vi "RunWireCalibration.vi"() -> ()   [LabVIEW 2016]
uses:
  Controls/0_XYZstage/BOOL_Moving.ctl
  <vilib>/userdefined/High Color/IMAQdx.ctl
  <vilib>/Utility/miscctls.llb/LVRowAndColumnUnsignedTypeDef.ctl
  Controls/All_Enums/Enum_TypeDef_ImageSharpnessAnalysisMethod.ctl
  <vilib>/Analysis/6fits.llb/Curve Fitting Criteria.ctl
  <extravilib>/ChannelInstances/High Speed Stream-c(i32,str,c(dbl,dbl),t'IMAQ Image.ctl',t'IMAQdx.ctl')/_Read For Replicate.vi
  Miscellaneous/PixelToMicron.vi
  <extravilib>/ChannelInstances/High Speed Stream-c(i32,str,c(dbl,dbl),t'IMAQ Image.ctl',t'IMAQdx.ctl')/Instantiate.vi
  <extravilib>/ChannelInstances/High Speed Stream-c(i32,str,c(dbl,dbl),t'IMAQ Image.ctl',t'IMAQdx.ctl')/)Channel.vi
  <extravilib>/ChannelInstances/High Speed Stream-c(i32,str,c(dbl,dbl),t'IMAQ Image.ctl',t'IMAQdx.ctl')/Abort Signal/Init Signal.vi
  <vilib>/gmath/statdist.llb/st_Percentiles (scalar).vi
  <vilib>/vision/driver/NI_Vision_Acquisition_Software.lvlib
  <vilib>/Analysis/NI_AALPro.lvlib
  <vilib>/Analysis/NI_AALBase.lvlib
  <vilib>/gmath/NI_Gmath.lvlib
  <vilib>/LabVIEW Interface for Arduino/LabVIEW Interface for Arduino.lvlib
  <extravilib>/ChannelInstances/High Speed Stream-c(i32,str,c(dbl,dbl),t'IMAQ Image.ctl',t'IMAQdx.ctl').lvlib
panel:
  out "completed":bool
  out "Loops":i32
  out "Image Data":T1(array[cluster])
  in  "Mode":enum16{"Run Calibration", "View Results"}(ring)
  out "Finished":bool
  in  "Tab Control":T2(tab)
  in  "error tab":bool
  in  "cam session":T3="cam1" caption="Select Camera"
  in  "Short-distance\naxis speed":T4={"vX [mm/s]"=5.0, "vY [mm/s]"=5.0, "vZ [mm/s]"=5.0}
  in  "Long-distance\naxis speed":T4={"vX [mm/s]"=25.0, "vY [mm/s]"=12.5, "vZ [mm/s]"=5.0}
  in  "wait time":u32=2000 caption="wait (ms)"
  in  "Y position":dbl format="%#_13g"
  in  "Z position":dbl format="%#_13g"
  in  "percentile":dbl=95.0 caption="tolerance percentile" format="%#_13g"
  in  "Python":path=path "python"
  in  "Wire Diameter":dbl=90.0 caption="Wire Diameter (microns)"
  in  "Wire Height (mm)":dbl=2.5 format="%#_13g"
  in  "Image Info Results Read":path caption="Image Info Path"
  in  "Image File Results Read":bool=TRUE caption="View Images from Saved Location?"
  in  "Im. Source":T5(radio)
  out "Image Source Tab":T5(tab) caption="Warning: if you don't save the images, a new set of images must be captured to run the calibration again. Saving images allows the user to run the calibration on the same image set multiple times."
  in  "Disable auto-focus":bool caption="(only use if the camera was not adjusted since the most recent run of this VI)"
  in  "Home":bool=TRUE caption="Home first?"
  in  "Save Images":bool=TRUE caption="Save Images to File?"
  in  "Image Calibration Write":path=path "C:/Users/Aerotech/Desktop/Joel Images 8_7" caption="Image Path"
  in  "Image Overwrite":bool=TRUE caption="Overwrite existing files?"
  in  "Image Info Calibration Read":path caption="Image Info Path"
  in  "View Results":bool
  in  "Data File Read":path caption="Data File Path"
  in  "Run Calibration":bool
  in  "File Name":string="data_file.csv"
  in  "Data File Overwrite":bool caption="Overwrite existing files?"
  in  "Data File Write":path=path "C:/Users/Aerotech/Desktop" caption="Data File Path"
  in  "List of All Fits":i32(listbox)
  out "Progress":dbl(slide) caption="Progress: complete" scale=0.0..100.0
  out "Moving":T6
  in  "abort":bool
  in  "pause":bool
  out "Graph of Fit":cluster{dbl[], dbl[]}[](graph) caption="Graph of Fit for Image #79"
  in  "List of Failed Fits":i32(listbox)
  out "Image":T7(plugin-control) caption="Image #79"
  out "Fit Info":T8={"Initial Guess"={"Center (pixels)"=-1.0, "Reflectivity"=0.0}, "Params Vector"=[], "Errors"=[], "Iterations"=0, "Success"=FALSE} {"Errors" format="%#_2g"; "Params Vector" format="%#_10f"; "Initial Guess"."Center (pixels)" format="%#_16g"}
  in  "Quit":bool
  out "Re-do Necessary?":bool
  out "fails":i32 caption="Number of Failed Fits:"
  out "Tolerance":dbl=4.0 caption="95% Tolerance (microns):" format="%_2g"
  out "Confidence":dbl caption="95% Confidence Interval (microns):" format="%.5g"
  out "std. dev.":dbl caption="Standard Deviation (microns):" format="%.5g"
  out "outside tolerance":bool caption="Within Tolerance?"
  out "Histogram of Final Fit Residuals":T9(graph) caption="XY Graph"
  out "Adjusted Graph of Final Fit":cluster{dbl[], dbl[]}(graph) caption="XY Graph"
  out "queue error":errorcluster
  out "image file error":errorcluster
  out "info file error":errorcluster
  out "Image Display Error":errorcluster
  out "data file write error":errorcluster
  out "Capture Error":errorcluster caption="stage/camera error"
  # "NOTE: Click \"RUN\" to run the VI BEFORE entering the set-up parameters!!!"
  # "For runnung a new calibration"
  # "For viewing a previously run calibration"
  # "Image Files"
  # "Settings"
  # "Image Files"
  # "Data File"
  # "Data File"
  # "Center (px)"
  # "Reflectivity (ul)"
  # "Amplitude (px val^2)"
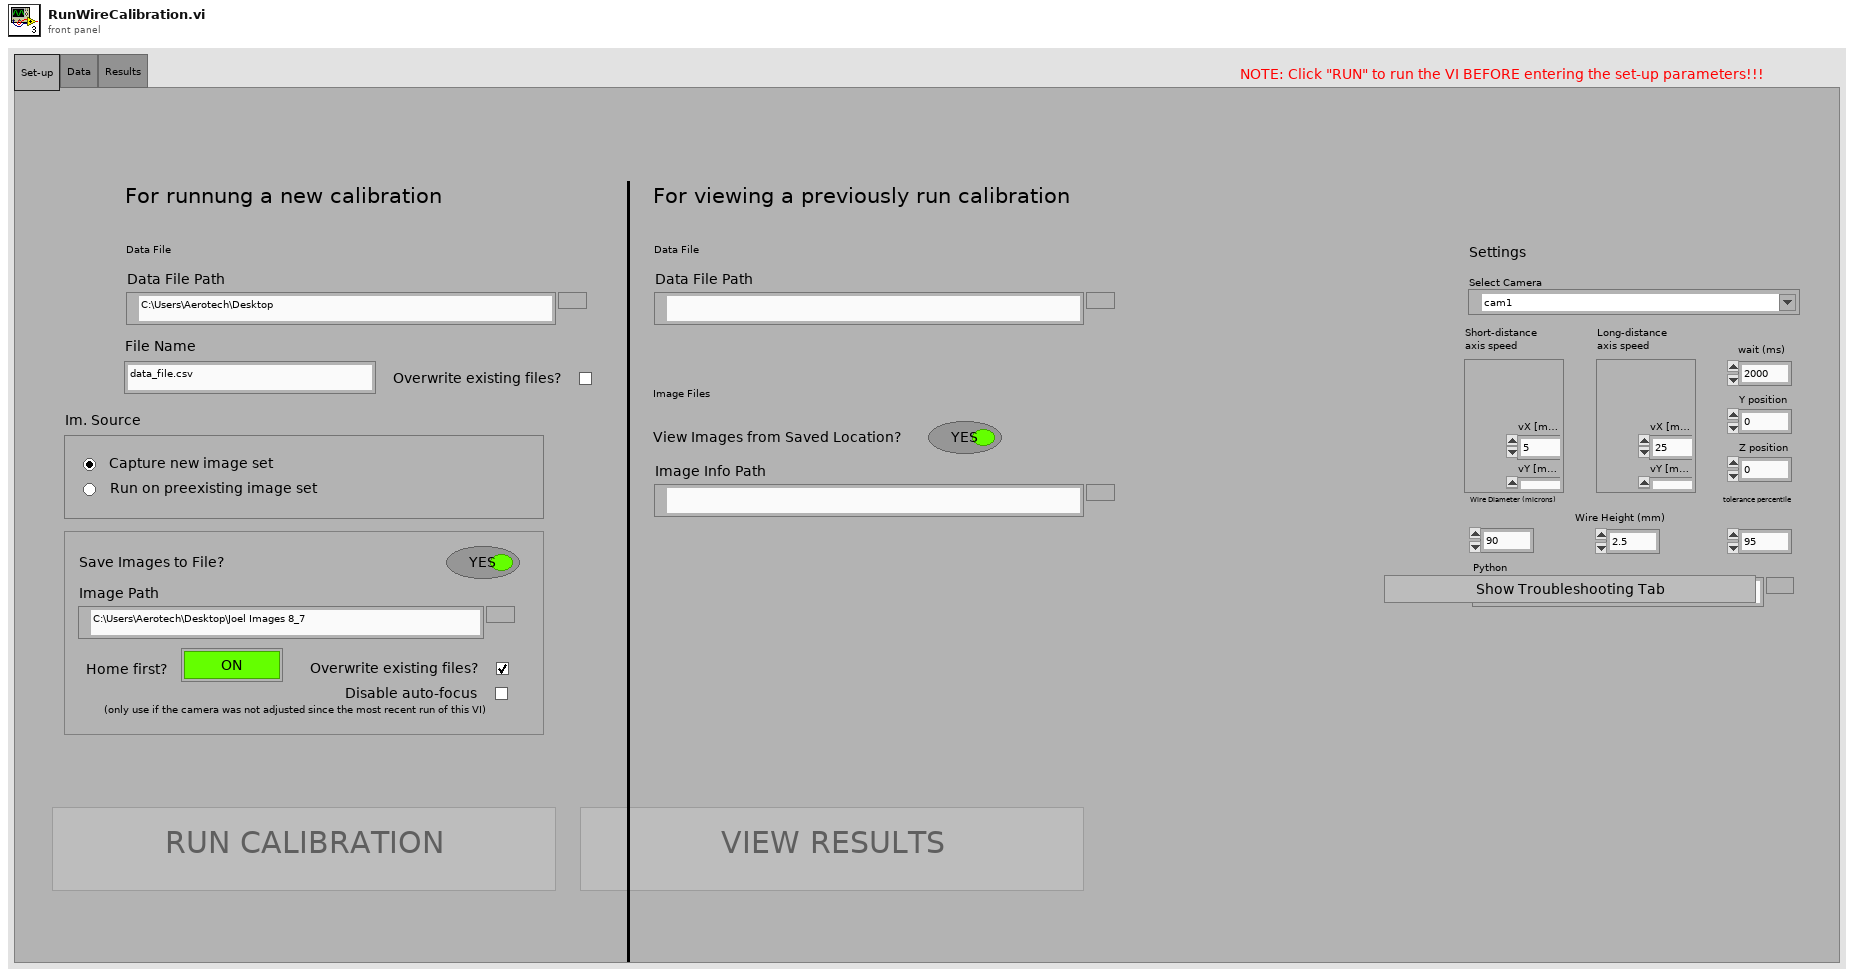
[diagram p1: front panel]
types:
  T1 = cluster{"success?":bool, "image number":i32, "camera position":cluster{"X":dbl, "Y":dbl}, "parameters":cluster{"amplitude":dbl, "center":dbl, "reflectivity":dbl}, "errors":cluster{"amplitude":dbl, "center":dbl, "reflectivity":dbl}, "Initial Guess":cluster{"center":dbl, "reflectivity":dbl}, "iterations":i32, "image path":path}[]
  T2 = enum32{"Set-up", "Data", "Results", "Troubleshooting"}
  T3 = typedef "IMAQdx.ctl" = refnum<k21>
  T4 = cluster{"vX [mm/s]":dbl, "vY [mm/s]":dbl, "vZ [mm/s]":dbl}
  T5 = enum32{"Capture new image set", "Run on preexisting image set"}
  T6 = typedef "BOOL_Moving.ctl" = bool
  T7 = typedef "IMAQ Image.ctl" = refnum<image>
  T8 = cluster{"Initial Guess":cluster{"Center (pixels)":dbl, "Reflectivity":dbl}, "Params Vector":dbl[], "Errors":dbl[], "Iterations":i32, "Success":bool}
  T9 = cluster{"X Values":dbl[], "Histogram: h(x)":i32[]}
  T10 = enum8{"Enabled", "Disabled", "Disabled and Grayed Out"}
  T11 = cluster{"Params Vector[1]":dbl, "Params Vector[2]":dbl}
  T12 = enum16{"open", "replace", "create", "open or create", "replace or create", "replace or create with confirmation"}
  T13 = cluster{"image number":i32, "image path":path, "position":cluster{dbl, dbl}}
  T14 = typedef "Enum_TypeDef_ImageSharpnessAnalysisMethod.ctl" = enum16{"sigma( Intensity )", "Mean( Laplacian Convolution )"}
  T15 = typedef "LVRowAndColumnUnsignedTypeDef.ctl" = cluster{"Row":u32, "Column":u32}
  T16 = cluster{"Data File Write":path, "File Name":string, "Data File Overwrite":bool}
  T17 = typedef "LabVIEW Interface for Arduino.lvlib/Arduino Resource.ctl" = cluster{"VISA resource":refnum<visa-resource-name>, "Board Type":T18, "Connection Type":enum8{"USB / Serial"}, "Bytes Per Packet (15)":u8}
  T18 = typedef "LabVIEW Interface for Arduino.lvlib/Board Type.ctl" = enum16{"Uno", "Dimuelanove w/Atmega 328", "Mega 2560"}
  T19 = typedef "ArduinoLT-ConfigurationControl.ctl" = cluster{"Lights: Digital I/O Pins":cluster{"Coaxial":u8, "Spotlights":u8}, "Thermistor Settings":cluster{"Analogue Readout Pin":u8, "Vcc Reference Pin":u8, "Paired Resistance (10K Ohms)":dbl, "Units (C)":enum16{"Celsius", "Fahrenheit", "Kelvin"}}}
  T20 = cluster{"Arduino Configuration OUT":T19, "Arduino Resource OUT":T17, "error out":errorcluster}
  T21 = typedef "Image Type" = u32
  T22 = cluster{"Final X":dbl, "Final Y":dbl, "Final Z":dbl}
  T23 = cluster{i32, string, cluster{"Final X":dbl, "Final Y":dbl}, "Image Out":T7, "Session Out":T3}
  T24 = typedef "High Speed Stream-c(i32,str,c(dbl,dbl),t'IMAQ Image.ctl',t'IMAQdx.ctl').lvlib/)Channel.ctl" = refnum<queue>
  T25 = cluster{"Image Calibration Write":path, "Image Overwrite":bool}
  T26 = cluster{i32, "Smart Path":path, cluster{"Final X":dbl, "Final Y":dbl}}
  T27 = cluster{i32, "appended path":path, cluster{dbl, dbl}}
  T28 = cluster{"Params Vector[0]":dbl, "Params Vector[1]":dbl, "Params Vector[2]":dbl}
  T29 = cluster{"Errors[0]":dbl, "Errors[1]":dbl, "Errors[2]":dbl}
  T30 = cluster{"Success":bool, "image number":i32, "position":cluster{dbl, dbl}, "Params Vector":cluster{"Params Vector[0]":dbl, "Params Vector[1]":dbl, "Params Vector[2]":dbl}, "Errors":cluster{"Errors[0]":dbl, "Errors[1]":dbl, "Errors[2]":dbl}, cluster{"Params Vector[1]":dbl, "Params Vector[2]":dbl}, "Iterations":i32, "image path":path}
  T31 = cluster{"Success":bool, "image number":i32, "position":cluster{"X":dbl, "Y":dbl}, "Params Vector":cluster{"Params Vector[0]":dbl, "Params Vector[1]":dbl, "Params Vector[2]":dbl}, "Errors":cluster{"Errors[0]":dbl, "Errors[1]":dbl, "Errors[2]":dbl}, "Initial Guess":cluster{"Params Vector[1]":dbl, "Params Vector[2]":dbl}, "Iterations":i32, "image path":path}[]
  T32 = cluster{bool, i32, cluster{dbl, dbl}, cluster{dbl, dbl, dbl}, cluster{dbl, dbl, dbl}, cluster{dbl, dbl}, i32, "appended path":path}
  T33 = typedef "NI_AALPro.lvlib/Curve Fitting Criteria.ctl" = u16
  T34 = cluster{"success?":bool, "image number":i32, "camera position":cluster{"X":dbl, "Y":dbl}, "parameters":cluster{"amplitude":dbl, "center":dbl, "reflectivity":dbl}, "errors":cluster{"amplitude":dbl, "center":dbl, "reflectivity":dbl}, "Initial Guess":cluster{"center":dbl, "reflectivity":dbl}, "iterations":i32, "image path":path}
  T35 = cluster{"amplitude":dbl, "center":dbl, "reflectivity":dbl}
  T36 = cluster{"Initial Guess":cluster{"center":dbl, "reflectivity":dbl}, "parameters":dbl[], "errors":dbl[], "iterations":i32, "success?":bool}
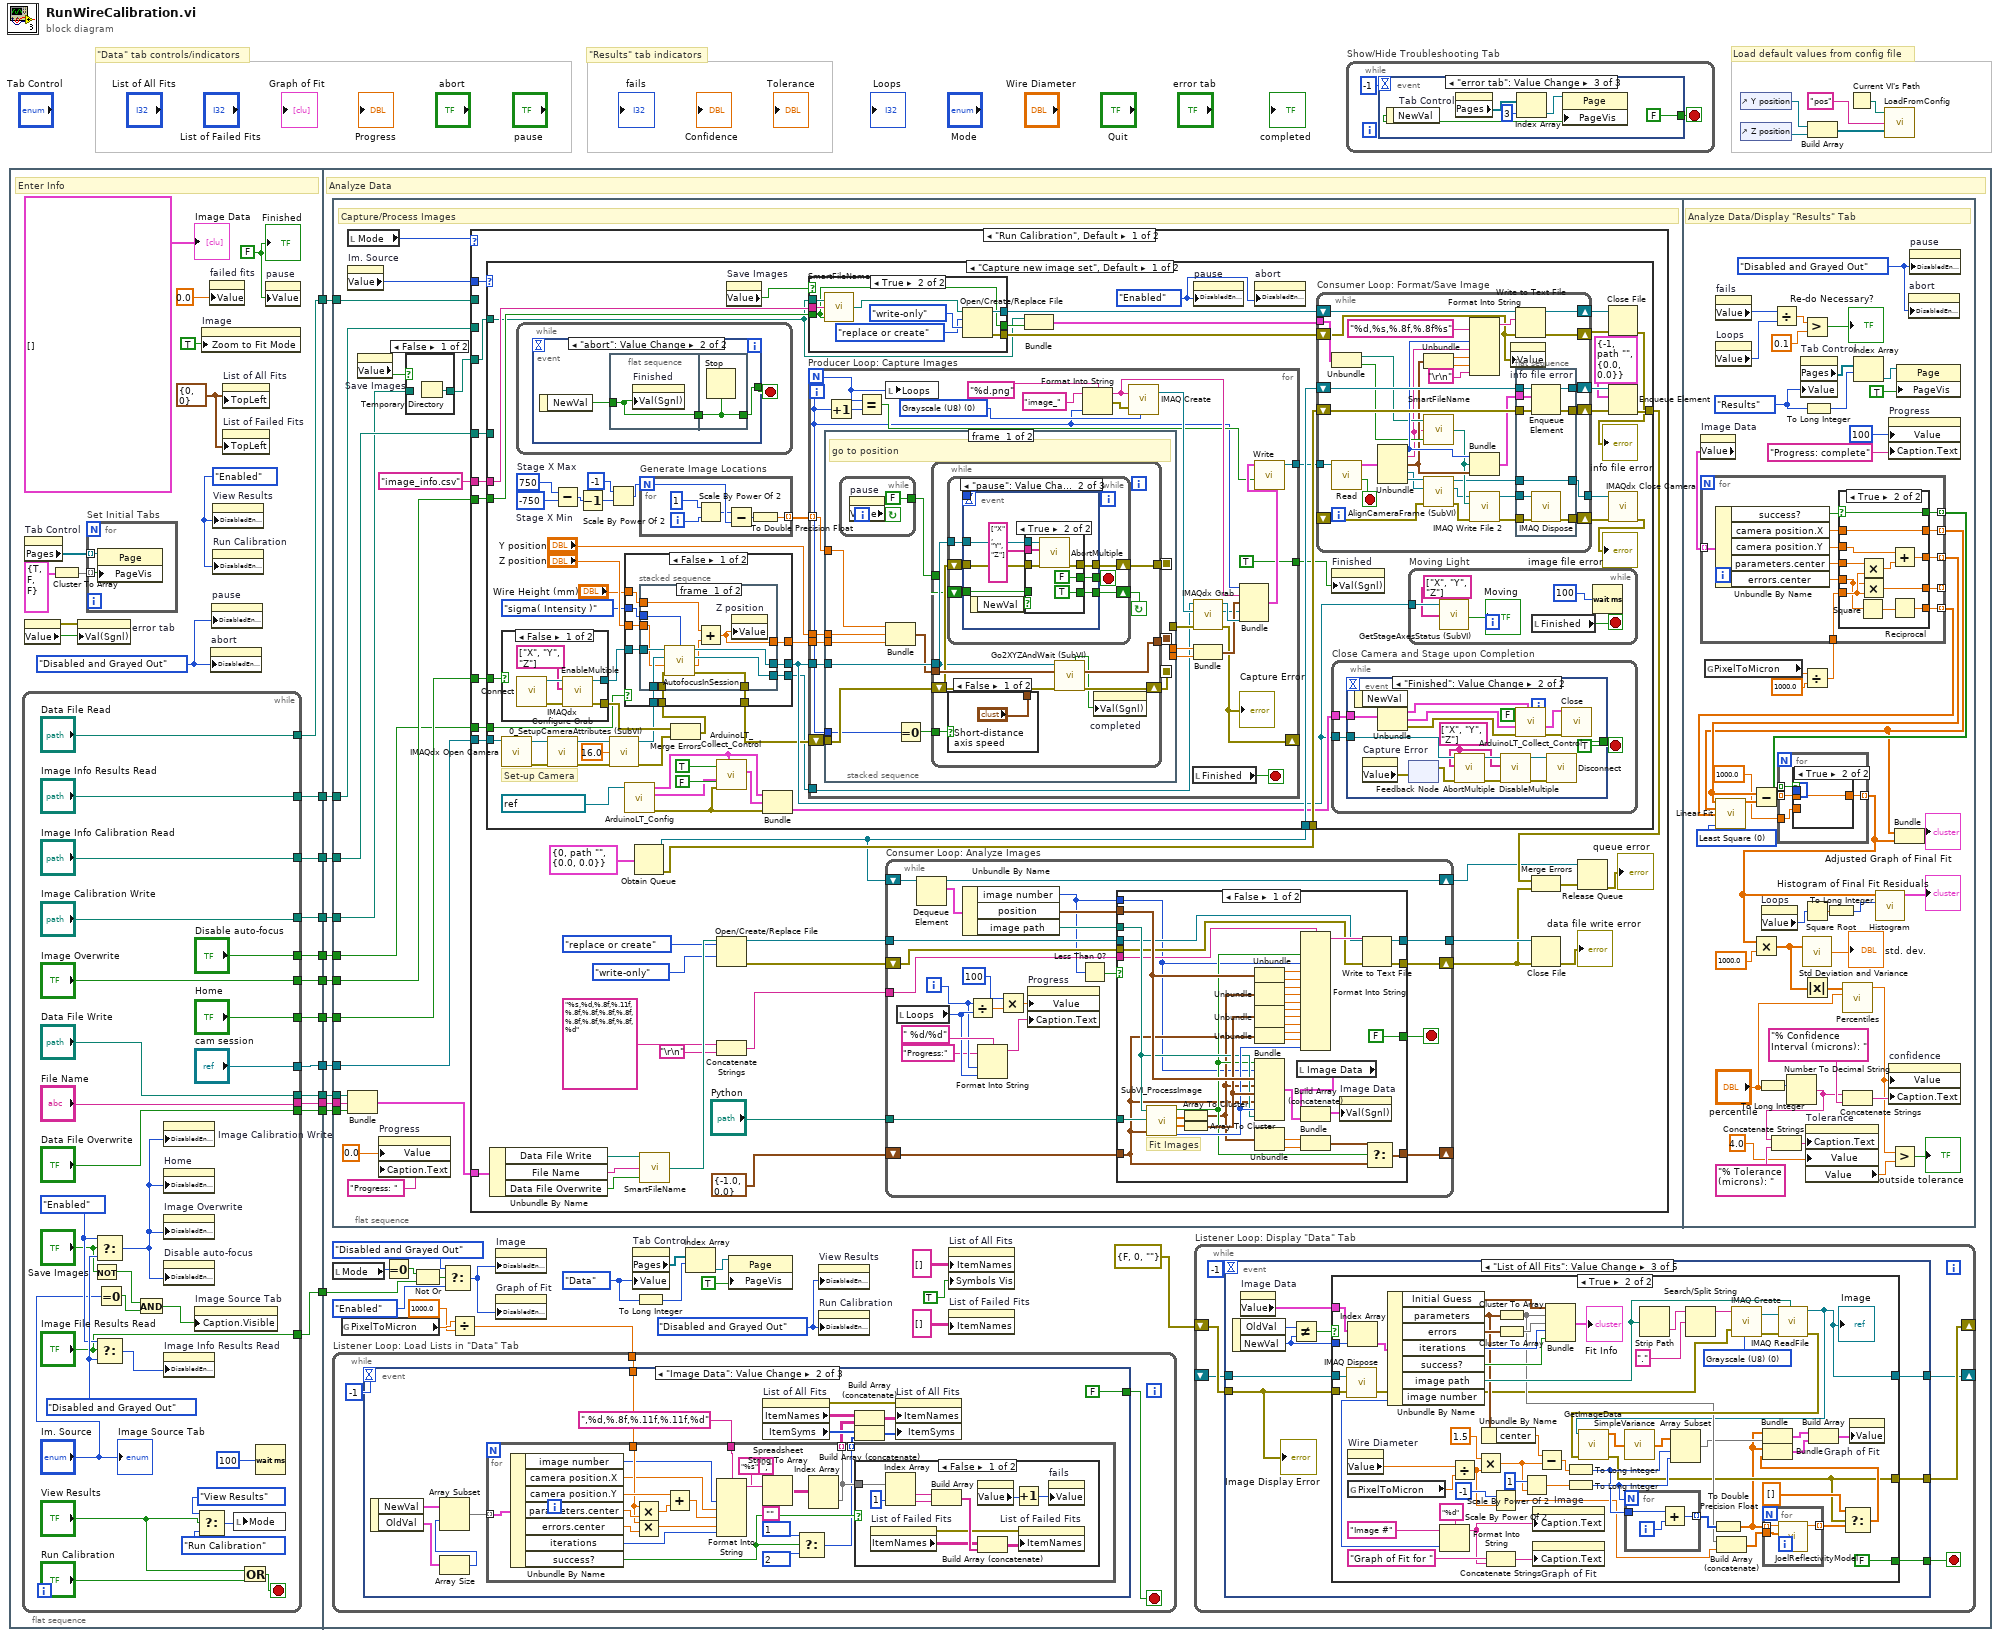
[diagram p0: block diagram]
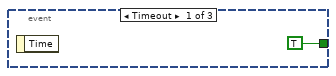
[diagram p2: hidden frame]
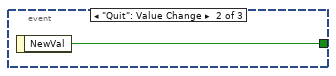
[diagram p3: hidden frame]
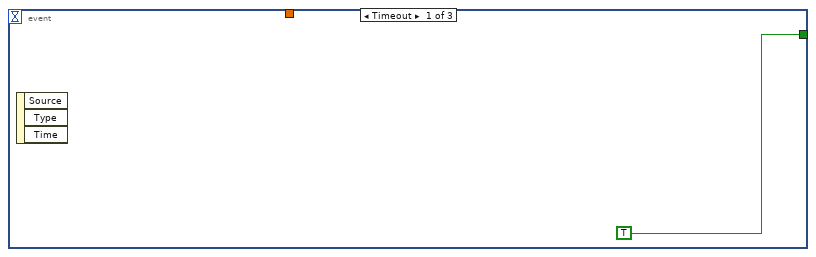
[diagram p4: hidden frame]
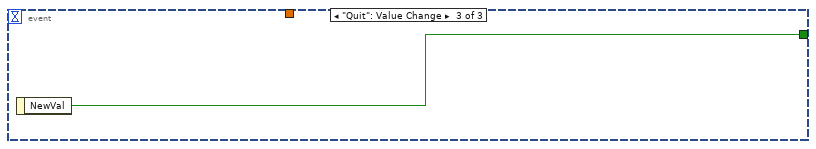
[diagram p6: hidden frame]
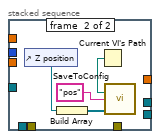
[diagram p8: hidden frame]
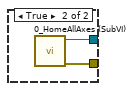
[diagram p10: hidden frame]
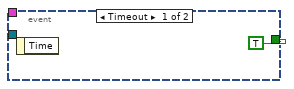
[diagram p11: hidden frame]
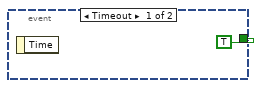
[diagram p12: hidden frame]
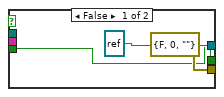
[diagram p13: hidden frame]
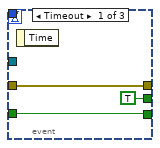
[diagram p14: hidden frame]
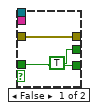
[diagram p15: hidden frame]
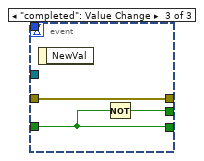
[diagram p16: hidden frame]
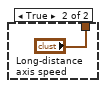
[diagram p17: hidden frame]
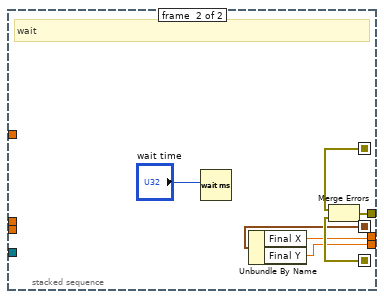
[diagram p18: hidden frame]
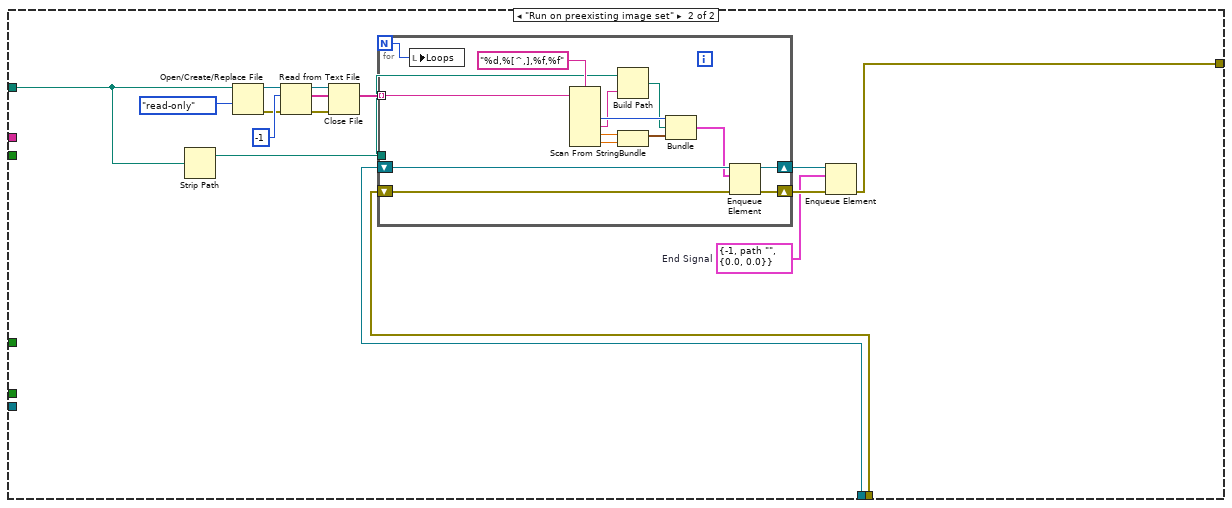
[diagram p19: hidden frame]
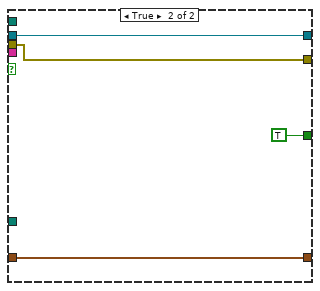
[diagram p20: hidden frame]
diagram:
  # "Load default values from config file"
  # "\"Results\" tab indicators"
  # "\"Data\" tab controls/indicators"
  n1 = flat-sequence {
    tunnel: [w32] -> w17
    tunnel: [w34] -> w16
    tunnel: [w40] -> w15
    tunnel: [w39] -> w14
    tunnel: [w38] -> w13
    tunnel: [w37] -> w12
    tunnel: [w36] -> w11
    tunnel: [w35] -> w10
    tunnel: [w33] -> w9
    tunnel: [w25] -> w8
    tunnel: [w22] -> w7
    tunnel: [w18] -> w6
    tunnel: w17 -> [w94]
    tunnel: w16 -> [w93]
    tunnel: w15 -> [w92]
    tunnel: w14 -> [w87]
    tunnel: w13 -> [w86]
    tunnel: w12 -> [w85]
    tunnel: w11 -> [w84]
    tunnel: w10 -> [w83]
    tunnel: w9 -> [w82]
    tunnel: w8 -> [w75]
    tunnel: w7 -> [w73]
    tunnel: w6 -> [w72]
    frame #0 {
      w21 = FALSE ("Finished")
      w23 = T10."Disabled and Grayed Out" ("Disabled")
      w24 = T10."Enabled" ("Disabled")
      w29 = T15 {"Row"=0, "Column"=0} ("Top Left Visible Cell")
      # "Enter Info"
      n2 = while {
        tunnel: ["Image Overwrite"] -> w40
        tunnel: ["Data File Write"] -> w39
        tunnel: ["File Name"] -> w38
        tunnel: ["Data File Overwrite"] -> w37
        tunnel: ["cam session"] -> w36
        tunnel: ["Image Calibration Write"] -> w35
        tunnel: ["Image Info Calibration Read"] -> w34
        tunnel: ["Image Info Results Read"] -> w33
        tunnel: ["Data File Read"] -> w32
        tunnel: ["Image File Results Read"] -> w25
        tunnel: ["Home"] -> w22
        tunnel: ["Disable auto-focus"] -> w18
        stop <- w60 stop-if-true
        w66 = T10."Enabled" ("Disabled")
        w67 = T10."Disabled and Grayed Out" ("Disabled")
        n3 = Not(x="Save Images") -> (.not. x?=w52:bool)
        n4 = Select(t=w66, s="Save Images", f=w67) -> (s? t:f=w44:T10)
        n5 = Select(t=w66, s="Image File Results Read", f=w67) -> (s? t:f=w54:T10)
        n6 = Equal To 0?(x="Im. Source") -> (x = 0?=w50:bool)
        n7 = And(x=w52, y=w50) -> (x .and. y?=w51:bool)
        n8 = property on="Image Calibration Write" class="Path"("DisabledEnum"=w44) -> ()  [unwired: 2 in, 2 out]
        n9 = property on="Home" class="Bool (strict)"("DisabledEnum"=w44) -> ()  [unwired: 2 in, 2 out]
        n10 = property on="Image Overwrite" class="Bool (strict)"("DisabledEnum"=w44) -> ()  [unwired: 2 in, 2 out]
        n11 = property on="Disable auto-focus" class="Bool (strict)"("DisabledEnum"=w44) -> ()  [unwired: 2 in, 2 out]
        n12 = property on="Image Info Results Read" class="Path"("DisabledEnum"=w54) -> ()  [unwired: 2 in, 2 out]
        n13 = property on="Image Source Tab" class="TabCtl (strict)"("Caption.Visible"=w51) -> ()  [unwired: 2 in, 2 out]
        n14 = Select(t=enum16{"Run Calibration", "View Results"}."View Results" ("Mode"), s="View Results", f=enum16{"Run Calibration", "View Results"}."Run Calibration" ("Mode")) -> (s? t:f=w65:enum16{"Run Calibration", "View Results"})
        n15 = local write "Mode"(w65) -> ()
        n16 = Or(x="View Results", y="Run Calibration") -> (x .or. y?=w60:bool)
        n17 = Wait (ms)(milliseconds to wait=u32 100) -> ()  [unwired: 1 out]
        "Image Source Tab" <- "Im. Source"
      }
      n18 = property on="Tab Control" class="TabCtl (strict)"() -> ("Pages"=w28:refnum<vi>[])  [unwired: 2 in, 2 out]
      n19 = property on="error tab" class="Bool (strict)"() -> (error out=w20:errorcluster, "Value"=w19:bool)  [unwired: 2 in, 1 out]
      n20 = Cluster To Array(cluster=cluster{bool, bool, bool} {TRUE, FALSE, FALSE}) -> (array=w26:bool[])
      n21 = property on="error tab" class="Bool (strict)"(error in=w20, "Val(Sgnl)"=w19) -> ()  [unwired: 1 in, 2 out]
      n22 = for "Set Initial Tabs" {
        tunnel: w28 -> [w43] mode=indexing
        tunnel: w26 -> [w42] mode=indexing
        n23 = property class="Page"(reference=w43, "PageVis"=w42) -> ()  [unwired: 1 in, 2 out]
      }
      n24 = property on="Image" class="ImageControl"("Zoom to Fit Mode"=TRUE) -> ()  [unwired: 2 in, 2 out]
      n25 = property on="failed fits" class="DigNum (strict)"("Value"=0.0 ("Number of Failed Fits:")) -> ()  [unwired: 2 in, 2 out]
      n26 = property on="abort" class="Bool"("DisabledEnum"=w23) -> ()  [unwired: 2 in, 2 out]
      n27 = property on="pause" class="Bool (strict)"("DisabledEnum"=w23) -> ()  [unwired: 2 in, 2 out]
      n28 = property on="View Results" class="Bool"("DisabledEnum"=w24) -> ()  [unwired: 2 in, 2 out]
      n29 = property on="Run Calibration" class="Bool"("DisabledEnum"=w24) -> ()  [unwired: 2 in, 2 out]
      n30 = property on="List of All Fits" class="MCListbox (strict)"("TopLeft"=w29) -> ()  [unwired: 2 in, 2 out]
      n31 = property on="List of Failed Fits" class="MCListbox (strict)"("TopLeft"=w29) -> ()  [unwired: 2 in, 2 out]
      n32 = property on="pause" class="Bool (strict)"("Value"=w21) -> ()  [unwired: 2 in, 2 out]
      "Image Data" <- T1 []
      "Finished" <- w21
    }
    frame #1 {
      w74 = T10."Disabled and Grayed Out" ("Disabled")
      w96 = T2."Data" ("Tab Control")
      # "Analyze Data"
      n33 = flat-sequence {
        tunnel: w94 -> [w170]
        tunnel: w93 -> [w159]
        tunnel: w92 -> [w169]
        tunnel: w87 -> [w167]
        tunnel: w86 -> [w166]
        tunnel: w85 -> [w165]
        tunnel: w84 -> [w163]
        tunnel: w83 -> [w157]
        tunnel: w82 -> [w162]
        tunnel: w73 -> [w155]
        tunnel: w72 -> [w154]
        frame #0 {
          # "Capture/Process Images"
          n34 = local read "Mode"() -> (w172:enum16{"Run Calibration", "View Results"})
          n35 = property on="Im. Source" class="RadioBtnsControl (strict)"() -> ("Value"=w171:T5)  [unwired: 2 in, 2 out]
          n36 = Bundle("Data File Write"=w167, "File Name"=w166, "Data File Overwrite"=w165) -> (w164:T16)  [unwired: 1 in]
          n37 = property on="Save Images" class="Bool (strict)"() -> ("Value"=w156:bool)  [unwired: 2 in, 2 out]
          n38 = property on="Progress" class="Slide (strict)"("Value"=0.0 ("Progress"), "Caption.Text"="Progress: ") -> ()  [unwired: 2 in, 2 out]
          n39 = case shown="False" w156 {
            tunnel: [w173 w174] -> w158
            tunnel: w157 -> [_ w174]
            frame False {
              n40 = Temporary Directory() -> (w173:path)
            }
            frame True {
            }
          }
          n41 = case shown="\"Run Calibration\", Default" w172 {
            tunnel: w171 -> [w205 _]
            tunnel: w164 -> [w199 _]
            tunnel: w170 -> [_ w589]
            tunnel: w162 -> [_ w583]
            tunnel: w159 -> [w198 _]
            tunnel: w163 -> [w197 _]
            tunnel: w169 -> [w196 _]
            tunnel: "image_info.csv" -> [w193 _]
            tunnel: w158 -> [w181 _]
            tunnel: w155 -> [w176 _]
            tunnel: w154 -> [w175 _]
            frame "Run Calibration", Default {
              n42 = Unbundle By Name(w199) -> ("Data File Write"=w179:path, "File Name"=w178:string, "Data File Overwrite"=w177:bool)
              n43 = Obtain Queue(element data type=T13 {"image number"=0, "image path"=path "", "position"={0.0, 0.0}} ("Cluster")) -> (queue out=w190:refnum<queue>, error out=w203:errorcluster)  [unwired: 4 in, 1 out]
              n44 = case shown="\"Capture new image set\", Default" w205 {
                tunnel: w203 -> [w239 w496]
                tunnel: w198 -> [_ w492]
                tunnel: w197 -> [w253 _]
                tunnel: w196 -> [w229 _]
                tunnel: w190 -> [w238 w497]
                tunnel: [w240 w486] -> w194
                tunnel: w193 -> [w227 _]
                tunnel: w181 -> [w222 _]
                tunnel: w176 -> [w220 _]
                tunnel: w175 -> [w219 _]
                frame "Capture new image set", Default {
                  w223 = T10."Enabled" ("Disabled")
                  w259 = 750  # Stage X Max
                  w258 = -750  # Stage X Min
                  # "Set-up Camera"
                  n45 = case shown="False" w220 {
                    tunnel: [w297 w300] -> w252
                    tunnel: [w296 w301] -> w217
                    frame False {
                      n46 = call "Connect.vi"() -> ("error out"=w299:errorcluster, "controller"=w298:refnum<k24>)  [unwired: 10 in]
                      n47 = call "EnableMultiple.vi"("error in (no error)"=w299, "axis names"=string[] ["X", "Y", "Z"], "controller in"=w298) -> ("error out"=w297:errorcluster, "controller out"=w296:refnum<k24>)  [unwired: 7 in]
                    }
                    frame True {
                      n48 = call "0_HomeAllAxes (SubVI).vi"() -> ("error out"=w300:errorcluster, "controller out"=w301:refnum<k24>)  [unwired: 8 in, 2 out]
                    }
                  }
                  n49 = call <vilib>:"IMAQdx Open Camera.vi"("Session In"=w253) -> ("error out"=w263:errorcluster, "Session Out"=w264:T3)  [unwired: 2 in, 7 out]
                  n50 = while {
                    stop <- w322 stop-if-true
                    n51 = event shown="[1] \"abort\": Value Change" {
                      selector: _ -> [_ _]
                      dyn-events: _ -> [_ _]
                      timeout: _ -> [_ _]
                      tunnel: [TRUE w324] -> w322
                      event Timeout {
                        n52 = event-data() -> ()  [unwired: 1 in, 1 out]
                      }
                      event "abort": Value Change {
                        n53 = event-data() -> ("NewVal"=w326:bool)  [unwired: 1 in]
                        n54 = flat-sequence {
                          tunnel: w326 -> [w327]
                          tunnel: [w327] -> w325
                          tunnel: w325 -> [w328]
                          tunnel: [w328] -> w324
                          frame #0 {
                            n55 = property on="Finished" class="Bool (strict)"("Val(Sgnl)"=w327) -> ()  [unwired: 2 in, 2 out]
                          }
                          frame #1 {
                            n56 = Stop(stop? (T)=w328) -> ()
                          }
                        }
                      }
                    }
                  }
                  n57 = call <vilib>:"IMAQdx Configure Grab.vi"("error in"=w263, "Session In"=w264) -> ("error out"=w261:errorcluster, "Session Out"=w262:T3)  [unwired: 8 out]
                  n58 = Subtract(x=w259, y=w258) -> (x-y=w257:i32)
                  n59 = Decrement(x=w257) -> (x-1=w256:i32)
                  n60 = Scale By Power Of 2(n=i8 -1, x=w256) -> (x*2^n=w254:i32)
                  n61 = call "0_SetupCameraAttributes (SubVI).vi"("error in (no error)"=w261, "Gain"=16.0, "Camera session in"=w262) -> ("error out"=w251:errorcluster, "Camera session out"=w214:T3)  [unwired: 7 in]
                  n62 = call "ArduinoLT_Config.vi"("VISA resource"=refnum<visa-resource-name> "LightsCTRL") -> ("error out"=w231:errorcluster, "Arduino Resource"=w248:T17, "Arduino Configuration OUT"=w221:T19)  [unwired: 4 in, 1 out]
                  n63 = for "Generate Image Locations" {
                    N: w254 -> [w481]
                    tunnel: [w478] -> w212 mode=indexing
                    i -> [w483]
                    n64 = Scale By Power Of 2(n=i8 1, x=w483) -> (x*2^n=w480:i32)
                    n65 = Subtract(x=w480, y=w481) -> (x-y=w479:i32)
                    n66 = To Double Precision Float(number=w479) -> (double precision float=w478:dbl)
                  }
                  n67 = Merge Errors(w252, w251) -> (w218:errorcluster)
                  n68 = case shown="False" w219 {
                    tunnel: w217 -> [w270 w294]
                    tunnel: w218 -> [w272 w293]
                    tunnel: w214 -> [w269 w292]
                    tunnel: [w275 w294] -> w216
                    tunnel: [w273 w293] -> w215
                    tunnel: [w274 w292] -> w213
                    tunnel: [w268 w291] -> w211
                    tunnel: "Z position" -> [w271 w291]
                    tunnel: "Wire Height (mm)" -> [w267 _]
                    tunnel: Enum_TypeDef_ImageSharpnessAnalysisMethod."sigma( Intensity )" ("Method") -> [w266 _]
                    frame False {
                      n69 = stacked-sequence {
                        tunnel: [w286 _] -> w275
                        tunnel: [w285 _] -> w274
                        tunnel: [w284 _] -> w273
                        tunnel: w272 -> [w283 _]
                        tunnel: w271 -> [w279 _]
                        tunnel: w270 -> [w282 _]
                        tunnel: w269 -> [w281 _]
                        tunnel: [w280 _] -> w268
                        tunnel: w267 -> [w277 _]
                        tunnel: w266 -> [w276 _]
                        frame #0 {
                          n70 = call "AutofocusInSession.vi"("Method"=w276, "controller in"=w282, "Session In"=w281, "Z position Guess"=w279, "error in (no error)"=w283) -> ("controller out"=w286:refnum<k24>, "Session Out"=w285:T3, "Autofocus Height"=w278:dbl, "error out"=w284:errorcluster)  [unwired: 1 out]
                          n71 = Add(x=w277, y=w278) -> (x+y=w280:dbl)
                          n72 = property on="Z position" class="DigNum (strict)"("Value"=w280) -> ()  [unwired: 2 in, 2 out]
                        }
                        frame #1 {
                          n73 = control-ref of="Z position"() -> (w288:refnum<vi>)
                          n74 = Build Array(w288) -> (w290:refnum<vi>[])
                          n75 = Current VI's Path() -> (path=w287:path)
                          n76 = call "SaveToConfig.vi"("Array"=w290, "Section"="pos", "VI Path"=w287) -> ()
                        }
                      }
                    }
                    frame True {
                    }
                  }
                  n77 = call "ArduinoLT_Collect_Control.vi"("Arduino Configuration"=w221, "error in"=w231, "Arduino Resource IN"=w248, "Spotlights"=FALSE, "Coaxial light"=TRUE) -> ("Arduino Resource OUT"=w232:T17)  [unwired: 4 in, 2 out]
                  n78 = property on="Save Images" class="Bool (strict)"() -> ("Value"=w247:bool)  [unwired: 2 in, 2 out]
                  n79 = Bundle("Arduino Configuration OUT"=w221, "Arduino Resource OUT"=w232, "error out"=w231) -> (w225:T20)  [unwired: 1 in]
                  n80 = case shown="True" w247 {
                    tunnel: w229 -> [w377 w381]
                    tunnel: [refnum<file> refnum ("refnum out") w386] -> w237
                    tunnel: [errorcluster {"status"=FALSE, "code"=0, "source"=""} ("error out") w385] -> w236
                    tunnel: w222 -> [_ w383]
                    tunnel: [w377 w381] -> w228
                    tunnel: w227 -> [_ w382]
                    frame False {
                    }
                    frame True {
                      n81 = call "SmartFileName.vi"("Allow Replacement (False)"=w381, "preferred name"=w382, "preferred path"=w383) -> ("Smart Path"=w380:path)
                      n82 = Open/Create/Replace File(file path (use dialog)=w380, operation (0:open)=T12."replace or create", access (0:read/write)=enum16{"read/write", "read-only", "write-only"}."write-only") -> (refnum out=w386:refnum<file>, error out=w385:errorcluster)  [unwired: 3 in, 1 out]
                    }
                  }
                  n83 = for "Producer Loop: Capture Images" {
                    N -> [w402]
                    tunnel: w213 -> [w394]
                    tunnel: w216 -> [w414]
                    tunnel: [TRUE] -> w230
                    shift-right: [w392] -> _
                    shift-left: w215 -> [w413]
                    tunnel: [w397] -> w224
                    tunnel: w212 -> [w390] mode=indexing
                    tunnel: w211 -> [w389]
                    tunnel: "Y position" -> [w388]
                    i -> [w393]
                    stop <- w396 stop-if-true
                    w410 = T21 0 items=["Grayscale (U8)", "Grayscale (I16)", "Grayscale (SGL)", "Complex (CSG)", "RGB (U32)", "HSL (U32)", "RGB (U64)", "Grayscale (U16)"] ("Image Type")
                    n84 = stacked-sequence {
                      seq-local: [w425 _] -> [_ w476]
                      seq-local: [w424 _] -> [_ w475]
                      seq-local: [w423 _] -> [_ w471]
                      tunnel: w414 -> [w422 _]
                      tunnel: w413 -> [w426 _]
                      tunnel: w393 -> [w416 _]
                      tunnel: [_ w472] -> w412
                      tunnel: [_ w474] -> w405
                      tunnel: [_ w473] -> w404
                      tunnel: w390 -> [w419 _]
                      tunnel: w389 -> [w418 _]
                      tunnel: w388 -> [w417 _]
                      frame #0 {
                        # "go to position"
                        n85 = while {
                          tunnel: [FALSE] -> w421
                          stop <- w428 continue-if-true
                          n86 = property on="pause" class="Bool (strict)"() -> ("Value"=w428:bool)  [unwired: 2 in, 2 out]
                        }
                        n87 = Bundle(w419, "Y position"=w417, "Z position"=w418) -> (w420:cluster{dbl, "Y position":dbl, "Z position":dbl})  [unwired: 1 in]
                        n88 = Equal To 0?(x=w416) -> (x = 0?=w415:bool)
                        n89 = while {
                          shift-right: [w437] -> w425
                          shift-left: w426 -> [w433]
                          tunnel: w420 -> [w438]
                          tunnel: [w436] -> w424
                          tunnel: [w432] -> w423
                          tunnel: w422 -> [w431]
                          tunnel: w421 -> [w430]
                          tunnel: w415 -> [w429]
                          stop <- w434 continue-if-true
                          n90 = while {
                            shift-right: [w444] -> w432
                            shift-left: w433 -> [w443]
                            shift-right: [w442] -> w434
                            shift-left: w430 -> [w441]
                            tunnel: w431 -> [w439]
                            stop <- w440 stop-if-true
                            n91 = event shown="[1] \"pause\": Value Change" {
                              selector: _ -> [_ _ _]
                              dyn-events: _ -> [_ _ _]
                              timeout: _ -> [w445 _ _]
                              tunnel: [w448 w456 w468] -> w444
                              tunnel: w443 -> [w448 w455 w468]
                              tunnel: [w447 w453 w466] -> w442
                              tunnel: w441 -> [w447 w452 w466]
                              tunnel: [TRUE ("NewVal") w451 w467] -> w440
                              tunnel: w439 -> [_ w449 _]
                              tunnel: [w445 _ _] -> _
                              event Timeout {
                                n92 = event-data() -> ()  [unwired: 1 in, 1 out]
                              }
                              event "pause": Value Change {
                                n93 = event-data() -> ("NewVal"=w454:bool)  [unwired: 1 in]
                                n94 = case shown="True" w454 {
                                tunnel: [w458 w465] -> w456
                                tunnel: string[] ["X", "Y", "Z"] ("axis names") -> [_ w464]
                                tunnel: w455 -> [w458 w463]
                                tunnel: [w459 TRUE] -> w453
                                tunnel: w452 -> [w459 _]
                                tunnel: [TRUE ("NewVal") FALSE ("NewVal")] -> w451
                                tunnel: w449 -> [_ w460]
                                frame False {
                                }
                                frame True {
                                n95 = call "AbortMultiple.vi"("error in (no error)"=w463, "axis names"=w464, "controller in"=w460) -> ("error out"=w465:errorcluster)  [unwired: 7 in, 1 out]
                                }
                                }
                              }
                              event "completed": Value Change {
                                n96 = event-data() -> ()  [unwired: 1 in, 1 out]
                                n97 = Not(x=w466) -> (.not. x?=w467:bool)
                              }
                            }
                          }
                          n98 = case shown="False" w429 {
                            tunnel: ["Short-distance\naxis speed" "Long-distance\naxis speed"] -> _
                            frame False {
                            }
                            frame True {
                            }
                          }
                          n99 = call "Go2XYZAndWait (SubVI).vi"(".NET Refnum in"=w431, "Go to Coordinates"=w438, "error in (no error)"=w433) -> ("completed"=w435:bool, "Final Position"=w436:T22, "error out"=w437:errorcluster)  [unwired: 8 in, 2 out]
                          n100 = property on="completed" class="Bool (strict)"("Val(Sgnl)"=w435) -> ()  [unwired: 2 in, 2 out]
                        }
                      }
                      frame #1 {
                        # "wait"
                        n101 = Wait (ms)(milliseconds to wait="wait time") -> ()  [unwired: 1 out]
                        n102 = Unbundle By Name(w475) -> ("Final X"=w473:dbl, "Final Y"=w474:dbl)
                        n103 = Merge Errors(w471, w476) -> (w472:errorcluster)
                      }
                    }
                    n104 = Increment(x=w393) -> (x+1=w403:i32)
                    n105 = Equal?(x=w402, y=w403) -> (x = y?=w398:bool)
                    n106 = local write "Loops"(w402) -> ()
                    n107 = Format Into String(format string="%d.png", initial string="image_", w393) -> (resulting string=w406:string, error out=w409:errorcluster)  [unwired: 1 in]
                    n108 = call "IMAQ Create"("Image Name"=w406, "Image Type"=w410, "error in (no error)"=w409) -> ("New Image"=w408:T7)  [unwired: 1 in, 2 out]
                    n109 = local read "Finished"() -> (w396:bool)
                    n110 = call <vilib>:"IMAQdx Grab.vi"("error in"=w412, "Image In"=w408, "Session In"=w394) -> ("error out"=w392:errorcluster, "Image Out"=w391:T7, "Session Out"=w401:T3)  [unwired: 1 in, 5 out]
                    "Capture Error" <- w392
                    n111 = Bundle("Final X"=w404, "Final Y"=w405) -> (w400:cluster{"Final X":dbl, "Final Y":dbl})  [unwired: 1 in]
                    n112 = Bundle(w393, w406, w400, "Image Out"=w391, "Session Out"=w401) -> (w399:T23)  [unwired: 1 in]
                    n113 = call <extravilib>:"Write.vi"("last element? (F)"=w398, "element"=w399) -> ("channel"=w397:T24)  [unwired: 7 in, 2 out]
                  }
                  n114 = Bundle("Image Calibration Write"=w222, "Image Overwrite"=w228) -> (w235:T25)  [unwired: 1 in]
                  n115 = property on="pause" class="Bool (strict)"("DisabledEnum"=w223) -> ()  [unwired: 2 in, 2 out]
                  n116 = property on="abort" class="Bool"("DisabledEnum"=w223) -> ()  [unwired: 2 in, 2 out]
                  n117 = while "Consumer Loop: Format/Save Image" {
                    tunnel: w224 -> [w337]
                    shift-right: [w358] -> w244
                    shift-left: w239 -> [w357]
                    shift-right: [w349] -> w246
                    shift-left: w236 -> [w329]
                    shift-right: [w348] -> w243
                    shift-left: w238 -> [w359]
                    shift-right: [w347] -> w245
                    shift-left: w237 -> [w350]
                    shift-right: [w360] -> w241
                    shift-left: _ -> [w344]
                    tunnel: w235 -> [w341]
                    tunnel: [w330] -> w234
                    stop <- w336 stop-if-true
                    n118 = Unbundle(w341) -> ("Image Calibration Write"=w342:path, "Image Overwrite"=w343:bool)
                    n119 = call <extravilib>:"Read.vi"("channel"=w337) -> ("done?"=w336:bool, "element"=w335:T23)  [unwired: 6 in, 3 out]
                    n120 = Unbundle(w335) -> (w355:i32, w332:string, w338:cluster{"Final X":dbl, "Final Y":dbl}, "Image Out"=w339:T7, "Session Out"=w340:T3)
                    n121 = Unbundle(w338) -> ("Final X"=w354:dbl, "Final Y"=w353:dbl)
                    n122 = call "SmartFileName.vi"("Allow Replacement (False)"=w343, "preferred name"=w332, "preferred path"=w342) -> ("Smart Path"=w334:path)
                    n123 = call "AlignCameraFrame (SubVI).vi"("error in (no error)"=w344, "Image Src"=w339, "Camera session in"=w340) -> ("error out"=w345:errorcluster, "Image Dst Out"=w333:T7, "Camera session out"=w331:T3)  [unwired: 6 in]
                    n124 = Format Into String(format string="%d,%s,%.8f,%.8f%s", w355, w332, w354, w353, "\r\n") -> (resulting string=w351:string)  [unwired: 2 in, 1 out]
                    n125 = Bundle(w355, "Smart Path"=w334, w338) -> (w356:T26)  [unwired: 1 in]
                    n126 = call-poly "IMAQ Write File 2"("error in (no error)"=w345, "File Path"=w334, "Image"=w333) -> ("error out"=w362:errorcluster, "Image Out (duplicate)"=w361:T7)  [unwired: 7 in]
                    n127 = property on="info file error" class="Clust (strict)"("Value"=w329) -> ()  [unwired: 2 in, 2 out]
                    n128 = Write to Text File(file (use dialog)=w350, text=w351, error in=w329) -> (refnum out=w347:refnum<file>, error out=w349:errorcluster)  [unwired: 1 in, 1 out]
                    n129 = flat-sequence {
                      tunnel: w362 -> [w371]
                      tunnel: w361 -> [w370]
                      tunnel: [w369] -> w360
                      tunnel: w359 -> [w368]
                      tunnel: [w367] -> w358
                      tunnel: w357 -> [w366]
                      tunnel: w356 -> [w365]
                      tunnel: [w364] -> w348
                      tunnel: w331 -> [w363]
                      tunnel: [w363] -> w330
                      frame #0 {
                        n130 = Enqueue Element(queue=w368, element=w365, error in (no error)=w366) -> (queue out=w364:refnum<queue>, error out=w367:errorcluster)  [unwired: 1 in, 1 out]
                        n131 = call "IMAQ Dispose"("Image"=w370, "error in (no error)"=w371) -> ("error out"=w369:errorcluster)  [unwired: 4 in]
                      }
                    }
                  }
                  n132 = property on="Finished" class="Bool (strict)"("Val(Sgnl)"=w230) -> ()  [unwired: 2 in, 2 out]
                  n133 = while "Close Camera and Stage upon Completion" {
                    tunnel: w225 -> [w303]
                    tunnel: w216 -> [w302]
                    stop <- w304 stop-if-true
                    n134 = event shown="[1] \"Finished\": Value Change" {
                      selector: _ -> [_ _]
                      dyn-events: _ -> [_ _]
                      timeout: _ -> [_ _]
                      tunnel: [TRUE TRUE] -> w304
                      tunnel: w303 -> [_ w318]
                      tunnel: w302 -> [_ w317]
                      event Timeout {
                        n135 = event-data() -> ()  [unwired: 1 in, 1 out]
                      }
                      event "Finished": Value Change {
                        w309 = FALSE ("Spotlights")
                        w315 = string[] ["X", "Y", "Z"] ("axis names")
                        n136 = event-data() -> ()  [unwired: 1 in, 1 out]
                        n137 = property on="Capture Error" class="Clust (strict)"() -> ("Value"=w313:errorcluster)  [unwired: 2 in, 2 out]
                        n138 = Unbundle(w318) -> ("Arduino Configuration OUT"=w306:T19, "Arduino Resource OUT"=w307:T17, "error out"=w308:errorcluster)
                        n139 = feedback-in #1(w313) -> ()
                        n140 = feedback #1() -> (w312:errorcluster)  [unwired: 1 in]
                        n141 = call "AbortMultiple.vi"("error in (no error)"=w312, "axis names"=w315, "controller in"=w317) -> ("error out"=w314:errorcluster, "controller out"=w316:refnum<k24>)  [unwired: 7 in]
                        n142 = call "DisableMultiple.vi"("error in (no error)"=w314, "axis names"=w315, "controller in"=w316) -> ("error out"=w320:errorcluster, "controller out"=w321:refnum<k24>)  [unwired: 7 in]
                        n143 = call "ArduinoLT_Collect_Control.vi"("Arduino Configuration"=w306, "error in"=w308, "Arduino Resource IN"=w307, "Spotlights"=w309, "Coaxial light"=w309) -> ("error out"=w310:errorcluster, "Arduino Resource OUT"=w311:T17)  [unwired: 4 in, 1 out]
                        n144 = call "Disconnect.vi"("error in (no error)"=w320, "controller"=w321) -> ()  [unwired: 9 in, 1 out]
                        n145 = call <vilib>:"Close.vi"("Arduino Resource"=w311, "error in"=w310) -> ()  [unwired: 13 in, 1 out]
                      }
                    }
                  }
                  n146 = while "Moving Light" {
                    tunnel: w216 -> [w375]
                    stop <- w372 stop-if-true
                    n147 = call "GetStageAxesStatus (SubVI).vi"(".NET Refnum in - Device"=w375, "Axes Names"=string[] ["X", "Y", "Z"] ("axis names")) -> ("Moving"=→"Moving":bool)  [unwired: 1 in, 7 out]
                    n148 = local read "Finished"() -> (w372:bool)
                    n149 = Wait (ms)(milliseconds to wait=u32 100) -> ()  [unwired: 1 out]
                  }
                  n150 = Close File(refnum=w245, error in=w246) -> (error out=→"info file error":errorcluster)  [unwired: 1 out]
                  n151 = Enqueue Element(queue=w243, element=T13 {"image number"=-1, "image path"=path "", "position"={0.0, 0.0}} ("End Signal"), error in (no error)=w244) -> (error out=w240:errorcluster)  [unwired: 1 in, 2 out]
                  n152 = call <vilib>:"IMAQdx Close Camera.vi"("error in"=w241, "Session In"=w234) -> ("error out"=→"image file error":errorcluster)  [unwired: 9 out]
                }
                frame "Run on preexisting image set" {
                  w484 = T13 {"image number"=-1, "image path"=path "", "position"={0.0, 0.0}}  # End Signal
                  n153 = Strip Path(path=w492) -> (stripped path=w493:path)  [unwired: 1 out]
                  n154 = Open/Create/Replace File(file path (use dialog)=w492, access (0:read/write)=enum16{"read/write", "read-only", "write-only"}."read-only") -> (refnum out=w491:refnum<file>, error out=w490:errorcluster)  [unwired: 4 in, 1 out]
                  n155 = Read from Text File(file (use dialog)=w491, count=-1, error in=w490) -> (refnum out=w488:refnum<file>, text=w494:string[], error out=w489:errorcluster)  [unwired: 1 in, 1 out]
                  n156 = Close File(refnum=w488, error in=w489) -> ()  [unwired: 2 out]
                  n157 = for {
                    N -> [w499]
                    shift-right: [w505] -> w487
                    shift-left: w496 -> [w512]
                    tunnel: w494 -> [w504] mode=indexing
                    tunnel: w493 -> [w503]
                    shift-right: [w500] -> w485
                    shift-left: w497 -> [w513]
                    n158 = local write "Loops"(w499) -> ()
                    n159 = Scan From String(format string="%d,%[^,],%f,%f", input string=w504) -> (output 1=w507:i32, output 2=w501:string, output 3=w510:dbl, output 4=w509:dbl)  [unwired: 6 in, 3 out]
                    n160 = Build Path(base path=w503, name or relative path=w501) -> (appended path=w502:path)
                    n161 = Bundle(w510, w509) -> (w508:cluster{dbl, dbl})  [unwired: 1 in]
                    n162 = Bundle(w507, "appended path"=w502, w508) -> (w506:T27)  [unwired: 1 in]
                    n163 = Enqueue Element(queue=w513, element=w506, error in (no error)=w512) -> (queue out=w500:refnum<queue>, error out=w505:errorcluster)  [unwired: 1 in, 1 out]
                  }
                  n164 = Enqueue Element(queue=w485, element=w484, error in (no error)=w487) -> (error out=w486:errorcluster)  [unwired: 1 in, 2 out]
                }
              }
              n165 = call "SmartFileName.vi"("Allow Replacement (False)"=w177, "preferred name"=w178, "preferred path"=w179) -> ("Smart Path"=w206:path)
              n166 = Open/Create/Replace File(file path (use dialog)=w206, operation (0:open)=T12."replace or create", access (0:read/write)=enum16{"read/write", "read-only", "write-only"}."write-only") -> (refnum out=w201:refnum<file>, error out=w180:errorcluster)  [unwired: 3 in, 1 out]
              n167 = Concatenate Strings("%s,%d,%.8f,%.11f,%.8f,%.8f,%.8f,%.8f,%.8f,%.8f,%.8f,%.8f,%d", "\r\n") -> (w184:string)
              n168 = while "Consumer Loop: Analyze Images" {
                shift-right: [w535] -> _
                shift-left: T11 {"Params Vector[1]"=-1.0, "Params Vector[2]"=0.0} -> [w525]
                tunnel: "Python" -> [w534]
                tunnel: w201 -> [w531]
                shift-right: [w530] -> w188
                shift-left: w180 -> [w529]
                tunnel: [w528] -> w200
                tunnel: w184 -> [w527]
                shift-right: [w526] -> w186
                shift-left: w190 -> [w537]
                i -> [w521]
                stop <- w514 stop-if-true
                n169 = local read "Loops"() -> (w522:i32)
                n170 = Dequeue Element(queue=w537) -> (queue out=w526:refnum<queue>, element=w536:T13)  [unwired: 2 in, 2 out]
                n171 = Unbundle By Name(w536) -> ("image number"=w516:i32, "position"=w533:cluster{dbl, dbl}, "image path"=w532:path)
                n172 = Divide(x=w521, y=w522) -> (x/y=w518:dbl)
                n173 = Format Into String(format string=" %d/%d", initial string="Progress:", w521, w522) -> (resulting string=w524:string)  [unwired: 1 in, 1 out]
                n174 = Multiply(x=100, y=w518) -> (x*y=w519:dbl)
                n175 = property on="Progress" class="Slide (strict)"("Value"=w519, "Caption.Text"=w524) -> ()  [unwired: 2 in, 2 out]
                n176 = Less Than 0?(x=w516) -> (x < 0?=w515:bool)
                n177 = case shown="False" w515 {
                  tunnel: [w570 w575] -> w535
                  tunnel: w534 -> [w569 _]
                  tunnel: w533 -> [w566 _]
                  tunnel: w532 -> [w553 _]
                  tunnel: w531 -> [w550 w574]
                  tunnel: [w549 w573] -> w530
                  tunnel: w529 -> [w548 w573]
                  tunnel: [w547 w574] -> w528
                  tunnel: w527 -> [w546 _]
                  tunnel: w525 -> [w540 w575]
                  tunnel: w516 -> [w539 _]
                  tunnel: [FALSE TRUE] -> w514
                  frame False {
                    # "Fit Images"
                    n178 = call "SubVI_ProcessImage.vi"("Image Path"=w553, "Path to Python.exe"=w569, "Initial Guess"=w540) -> ("Success"=w552:bool, "Params Vector"=w572:dbl[], "Errors"=w568:dbl[], "Iterations"=w554:i32)
                    n179 = Array To Cluster(array=w572) -> (cluster=w544:T28)
                    n180 = Array To Cluster(array=w568) -> (cluster=w565:T29)
                    n181 = Unbundle(w566) -> (w564:dbl, w563:dbl)
                    n182 = Unbundle(w544) -> ("Params Vector[0]"=w562:dbl, "Params Vector[1]"=w561:dbl, "Params Vector[2]"=w560:dbl)
                    n183 = Unbundle(w565) -> ("Errors[0]"=w559:dbl, "Errors[1]"=w558:dbl, "Errors[2]"=w557:dbl)
                    n184 = Unbundle(w540) -> ("Params Vector[1]"=w556:dbl, "Params Vector[2]"=w555:dbl)
                    n185 = Bundle("Success"=w552, "image number"=w539, "position"=w566, "Params Vector"=w544, "Errors"=w565, w540, "Iterations"=w554, "image path"=w553) -> (w567:T30)  [unwired: 1 in]
                    n186 = Unbundle(w544) -> ("Params Vector[1]"=w543:dbl, "Params Vector[2]"=w542:dbl)  [unwired: 1 out]
                    n187 = local read "Image Data"() -> (w571:T1)
                    n188 = Format Into String(format string=w546, w552, w539, w564, w563, w562, w561, w560, w559, w558, w557, w556, w555, w554) -> (resulting string=w551:string)  [unwired: 2 in, 1 out]
                    n189 = Build Array (concatenate)(w571, w567) -> (w545:T31)
                    n190 = Bundle("Params Vector[1]"=w543, "Params Vector[2]"=w542) -> (w541:T11)  [unwired: 1 in]
                    n191 = property on="Image Data" class="Arr (strict)"("Val(Sgnl)"=w545) -> ()  [unwired: 2 in, 2 out]
                    n192 = Write to Text File(file (use dialog)=w550, text=w551, error in=w548) -> (refnum out=w547:refnum<file>, error out=w549:errorcluster)  [unwired: 1 in, 1 out]
                    n193 = Select(t=w541, s=w552, f=w540) -> (s? t:f=w570:T11)
                  }
                  frame True {
                  }
                }
              }
              n194 = Merge Errors(w194, w188) -> (w189:errorcluster)
              n195 = Close File(refnum=w200, error in=w188) -> (error out=→"data file write error":errorcluster)  [unwired: 1 out]
              n196 = Release Queue(queue=w186, error in (no error)=w189) -> (error out=→"queue error":errorcluster)  [unwired: 1 in, 2 out]
            }
            frame "View Results" {
              n197 = property on="Image File Results Read" class="Bool (strict)"() -> ("Value"=w584:bool)  [unwired: 2 in, 2 out]
              n198 = Open/Create/Replace File(file path (use dialog)=w589, access (0:read/write)=enum16{"read/write", "read-only", "write-only"}."read-only") -> (refnum out=w588:refnum<file>, error out=w587:errorcluster)  [unwired: 4 in, 1 out]
              n199 = case shown="True" w584 {
                tunnel: w583 -> [_ w599]
                tunnel: [path "" w598] -> w582
                tunnel: [errorcluster {"status"=FALSE, "code"=0, "source"=""} ("error out") w596] -> w579
                tunnel: [string[] [] w593] -> w580
                frame False {
                }
                frame True {
                  n200 = Strip Path(path=w599) -> (stripped path=w598:path)  [unwired: 1 out]
                  n201 = Open/Create/Replace File(file path (use dialog)=w599, access (0:read/write)=enum16{"read/write", "read-only", "write-only"}."read-only") -> (refnum out=w595:refnum<file>, error out=w597:errorcluster)  [unwired: 4 in, 1 out]
                  n202 = Read from Text File(file (use dialog)=w595, count=-1, error in=w597) -> (text=w593:string[], error out=w596:errorcluster)  [unwired: 1 in, 2 out]
                }
              }
              n203 = Read from Text File(file (use dialog)=w588, count=-1, error in=w587) -> (text=w585:string[])  [unwired: 1 in, 3 out]
              n204 = for {
                N -> [w601]
                tunnel: w585 -> [w629] mode=indexing
                tunnel: "%[^,],%d,%f,%f,%f,%f,%f,%f,%f,%f,%f,%f,%d" -> [w612]
                tunnel: w584 -> [w606]
                tunnel: w582 -> [w605]
                tunnel: w580 -> [w604]
                tunnel: w579 -> [w602]
                tunnel: [w613] -> w577 mode=indexing
                i -> [w603]
                n205 = case shown="True" w606 {
                  tunnel: [path "" w635] -> w607
                  tunnel: w605 -> [_ w636]
                  tunnel: w604 -> [_ w638]
                  tunnel: w603 -> [_ w637]
                  tunnel: w602 -> [_ w634]
                  frame False {
                  }
                  frame True {
                    n206 = Index Array(array=w638, index=w637) -> (element=w631:string)
                    n207 = Scan From String(format string="%d,%[^,],", input string=w631, error in=w634) -> (output 2=w632:string)  [unwired: 4 in, 3 out]
                    n208 = Build Path(base path=w636, name or relative path=w632) -> (appended path=w635:path)
                  }
                }
                n209 = Scan From String(format string=w612, input string=w629) -> (output 1=w609:string, output 2=w618:i32, output 3=w628:dbl, output 4=w627:dbl, output 5=w626:dbl, output 6=w625:dbl, output 7=w624:dbl, output 8=w623:dbl, output 9=w622:dbl, output 10=w621:dbl, output 11=w620:dbl, output 12=w619:dbl, output 13=w611:i32)  [unwired: 15 in, 3 out]
                n210 = Bundle(w628, w627) -> (w617:cluster{dbl, dbl})  [unwired: 1 in]
                n211 = Bundle(w626, w625, w624) -> (w614:cluster{dbl, dbl, dbl})  [unwired: 1 in]
                n212 = Bundle(w623, w622, w621) -> (w616:cluster{dbl, dbl, dbl})  [unwired: 1 in]
                n213 = Bundle(w620, w619) -> (w615:cluster{dbl, dbl})  [unwired: 1 in]
                n214 = Type Cast(type=FALSE, x=w609) -> (*(type *) &x=w608:bool)
                n215 = property on="Loops" class="DigNum (strict)"("Value"=w601) -> ()  [unwired: 2 in, 2 out]
                n216 = Bundle(w608, w618, w617, w614, w616, w615, w611, "appended path"=w607) -> (w613:T32)  [unwired: 1 in]
              }
              n217 = property on="Image Data" class="Arr (strict)"("Val(Sgnl)"=w577) -> ()  [unwired: 2 in, 2 out]
            }
          }
        }
        frame #1 {
          w645 = T10."Disabled and Grayed Out" ("Disabled")
          w677 = T33 0 items=["Least Square", "Least Absolute Residual", "Bisquare"] ("method")
          w681 = T2."Results" ("Tab Control")
          # "Analyze Data/Display \"Results\" Tab"
          n218 = property on="Image Data" class="Arr (strict)"() -> ("Value"=w676:T1)  [unwired: 2 in, 2 out]
          n219 = global read "PixelToMicron.vi" "PixelToMicron"() -> (w675:dbl)
          n220 = property on="fails" class="DigNum (strict)"() -> ("Value"=w649:i32)  [unwired: 2 in, 2 out]
          n221 = property on="Loops" class="DigNum (strict)"() -> ("Value"=w648:i32)  [unwired: 2 in, 2 out]
          n222 = To Long Integer(number="percentile") -> (32bit integer=w664:i32)
          n223 = property on="Loops" class="DigNum (strict)"() -> ("Value"=w661:i32)  [unwired: 2 in, 2 out]
          n224 = Divide(x=w649, y=w648) -> (x/y=w650:dbl)
          n225 = Number To Decimal String(number=w664) -> (decimal integer string=w652:string)  [unwired: 1 in]
          n226 = Concatenate Strings(w652, "% Tolerance (microns): ") -> (w654:string)
          n227 = property on="Tab Control" class="TabCtl (strict)"("Value"=w681) -> ("Pages"=w682:refnum<vi>[])  [unwired: 2 in, 2 out]
          n228 = Greater?(x=w650, y=0.1) -> (0:→"Re-do Necessary?":bool)
          n229 = Divide(x=w675, y=1000.0) -> (x/y=w673:dbl)
          n230 = for {
            tunnel: w676 -> [w703] mode=indexing
            tunnel: w673 -> [w702]
            tunnel: [w696] -> w668 mode=indexing
            tunnel: [w695] -> w671 mode=indexing
            tunnel: [w694] -> _ mode=indexing
            tunnel: [w693] -> w646 mode=indexing
            tunnel: [w692] -> w669 mode=indexing
            n231 = Unbundle By Name(w703) -> ("success?"=w701:bool, "camera position.X"=w700:dbl, "camera position.Y"=w699:dbl, "parameters.center"=w698:dbl, "errors.center"=w697:dbl)
            n232 = case shown="True" w701 {
              selector: w701 -> [w705 w708]
              tunnel: w702 -> [_ w716]
              tunnel: w700 -> [w706 w713]
              tunnel: w699 -> [_ w714]
              tunnel: w698 -> [_ w717]
              tunnel: w697 -> [_ w710]
              tunnel: [w706 w713] -> w696
              tunnel: [w704 w712] -> w695
              tunnel: [w704 w711] -> w694
              tunnel: [w704 w707] -> w693
              tunnel: [w705 w708] -> w692
              frame False {
                w704 = 0.0
              }
              frame True {
                n233 = Square(x=w710) -> (x^2=w709:dbl)
                n234 = Multiply(x=w717, y=w716) -> (x*y=w715:dbl)
                n235 = Multiply(x=w710, y=w716) -> (x*y=w711:dbl)
                n236 = Add(x=w714, y=w715) -> (x+y=w712:dbl)
                n237 = Reciprocal(x=w709) -> (1/x=w707:dbl)
              }
            }
          }
          n238 = call <vilib>:"Linear Fit.vi"("Y"=w671, "X"=w668, "Weight"=w646, "method"=w677) -> ("Best Linear Fit"=w672:dbl[])  [unwired: 7 in, 4 out]
          n239 = Subtract(x=w671, y=w672) -> (x-y=w670:dbl[])
          n240 = for {
            tunnel: w670 -> [w688] mode=indexing
            tunnel: w669 -> [w689] mode=indexing
            tunnel: [w687] -> w657 mode=indexing
            tunnel: 1000.0 -> [w685]
            i -> [w686]
            n241 = case shown="True" w689 {
              tunnel: w688 -> [_ w691]
              tunnel: [0.0 w691] -> w687
              tunnel: w686 -> [_ _]
              tunnel: w685 -> [_ _]
              frame False {
              }
              frame True {
              }
            }
          }
          n242 = Multiply(x=w657, y=1000.0) -> (x*y=w656:dbl[])
          n243 = Square Root(x=w661) -> (sqrt(x)=w660:dbl)
          n244 = call <vilib>:"Std Deviation and Variance.vi"("X"=w656) -> ("standard deviation"=→"std. dev.":dbl)  [unwired: 1 in, 2 out]
          n245 = Absolute Value(x=w656) -> (abs(x)=w665:dbl[])
          n246 = To Long Integer(number=w681) -> (32bit integer=w680:i32)
          n247 = property on="Tolerance" class="DigNum (strict)"("Caption.Text"=w654, "Value"=4.0 ("Tolerance")) -> ("Value"=w641:dbl)  [unwired: 2 in, 2 out]
          n248 = To Long Integer(number=w660) -> (32bit integer=w659:i32)
          n249 = call-poly <vilib>:"Percentiles.vi"("p"="percentile", "x array"=w665) -> ("percentile"=w651:dbl)  [unwired: 8 in, 1 out]
          n250 = Concatenate Strings(w652, "% Confidence Interval (microns): ") -> (w663:string)
          n251 = Index Array(array=w682, index=w680) -> (element=w684:refnum<vi>)
          n252 = call <vilib>:"Histogram.vi"("intervals"=w659, "X"=w657) -> ("Histogram Graph"=→"Histogram of Final Fit Residuals":T9)  [unwired: 6 in, 3 out]
          n253 = property on="Progress" class="Slide (strict)"("Value"=u8 100 ("Progress"), "Caption.Text"="Progress: complete") -> ()  [unwired: 2 in, 2 out]
          n254 = property on="confidence" class="DigNum (strict)"("Value"=w651, "Caption.Text"=w663) -> ()  [unwired: 2 in, 2 out]
          n255 = Greater?(x=w651, y=w641) -> (0:→"outside tolerance":bool)
          n256 = Bundle(w668, w657) -> (→"Adjusted Graph of Final Fit":cluster{dbl[], dbl[]})  [unwired: 1 in]
          n257 = property class="Page"(reference=w684, "PageVis"=TRUE ("Page Visible")) -> ()  [unwired: 1 in, 2 out]
          n258 = property on="abort" class="Bool"("DisabledEnum"=w645) -> ()  [unwired: 2 in, 2 out]
          n259 = property on="pause" class="Bool (strict)"("DisabledEnum"=w645) -> ()  [unwired: 2 in, 2 out]
        }
      }
      n260 = local read "Mode"() -> (w78:enum16{"Run Calibration", "View Results"})
      n261 = global read "PixelToMicron.vi" "PixelToMicron"() -> (w99:dbl)
      n262 = Equal To 0?(x=w78) -> (x = 0?=w76:bool)
      n263 = Not Or(1:w75, 2:w76) -> (0:w77:bool)
      n264 = Select(t=T10."Disabled and Grayed Out" ("Disabled"), s=w77, f=T10."Enabled" ("Disabled")) -> (s? t:f=w80:T10)
      n265 = Divide(x=w99, y=1000.0) -> (x/y=w97:dbl)
      n266 = while "Listener Loop: Load Lists in \"Data\" Tab" {
        tunnel: w97 -> [w105]
        stop <- w104 stop-if-true
        n267 = event shown="[1] \"Image Data\": Value Change" {
          selector: _ -> [_ _ _]
          dyn-events: _ -> [_ _ _]
          timeout: -1 -> [_ _ _]
          tunnel: w105 -> [_ w120 _]
          tunnel: [TRUE FALSE w153] -> w104
          event Timeout {
            n268 = event-data() -> ()  [unwired: 1 in, 3 out]
          }
          event "Image Data": Value Change {
            n269 = event-data() -> ("NewVal"=w119:T1, "OldVal"=w118:T1)  [unwired: 1 in]
            n270 = Array Size(array=w118) -> (size(s)=w117:i32)
            n271 = Array Subset(array=w119, index=w117) -> (w116:T1)  [unwired: 1 in]
            n272 = for {
              tunnel: w120 -> [w138]
              tunnel: w116 -> [w125] mode=indexing
              tunnel: [w123] -> w110 mode=indexing
              tunnel: [w122] -> w109 mode=indexing
              tunnel: ",%d,%.8f,%.11f,%.11f,%d" -> [w121]
              n273 = Unbundle By Name(w125) -> ("image number"=w137:i32, "camera position.X"=w136:dbl, "camera position.Y"=w139:dbl, "parameters.center"=w141:dbl, "errors.center"=w142:dbl, "iterations"=w133:i32, "success?"=w124:bool)
              n274 = Multiply(x=w138, y=w141) -> (x*y=w140:dbl)
              n275 = Multiply(x=w138, y=w142) -> (x*y=w134:dbl)
              n276 = Add(x=w139, y=w140) -> (x+y=w135:dbl)
              n277 = Format Into String(format string=w121, w137, w136, w135, w134, w133) -> (resulting string=w132:string)  [unwired: 2 in, 1 out]
              n278 = Spreadsheet String To Array(delimiter (Tab)=",", format string="%s", spreadsheet string=w132, array type (2D Dbl)="") -> (array=w127:string[][])
              n279 = Select(t=1, s=w124, f=2) -> (s? t:f=w122:i32)
              n280 = Index Array(array=w127) -> (element=w123:string[])  [unwired: 2 in]
              n281 = case shown="False" w124 {
                tunnel: w123 -> [w151 _]
                frame False {
                  n282 = property on="List of Failed Fits" class="MCListbox (strict)"() -> (error out=w145:errorcluster, "ItemNames"=w146:string[][])  [unwired: 2 in, 1 out]
                  n283 = Index Array(array=w151, index #1=1) -> (element #1=w150:string, element #2=w149:string)  [unwired: 1 in]
                  n284 = Build Array(w150, w149) -> (w147:string[])
                  n285 = property on="fails" class="DigNum (strict)"() -> ("Value"=w144:i32)  [unwired: 2 in, 2 out]
                  n286 = Build Array (concatenate)(w146, w147) -> (w148:string[][])
                  n287 = Increment(x=w144) -> (x+1=w143:i32)
                  n288 = property on="List of Failed Fits" class="MCListbox (strict)"(error in=w145, "ItemNames"=w148) -> ()  [unwired: 1 in, 2 out]
                  n289 = property on="fails" class="DigNum (strict)"("Value"=w143) -> ()  [unwired: 2 in, 2 out]
                }
                frame True {
                }
              }
            }
            n290 = property on="List of All Fits" class="MCListbox (strict)"() -> (error out=w113:errorcluster, "ItemNames"=w114:string[][], "ItemSyms"=w112:i32[])  [unwired: 2 in, 1 out]
            n291 = Build Array (concatenate)(w114, w110) -> (w108:string[][])
            n292 = Build Array (concatenate)(w112, w109) -> (w111:i32[])
            n293 = property on="List of All Fits" class="MCListbox (strict)"(error in=w113, "ItemNames"=w108, "ItemSyms"=w111) -> ()  [unwired: 1 in, 2 out]
          }
          event "Quit": Value Change {
            n294 = event-data() -> ("NewVal"=w153:bool)  [unwired: 1 in]
          }
        }
      }
      n295 = property on="Image" class="ImageControl"("DisabledEnum"=w80) -> ()  [unwired: 2 in, 2 out]
      n296 = property on="Graph of Fit" class="XYGraph (strict)"("DisabledEnum"=w80) -> ()  [unwired: 2 in, 2 out]
      n297 = property on="Tab Control" class="TabCtl (strict)"("Value"=w96) -> ("Pages"=w100:refnum<vi>[])  [unwired: 2 in, 2 out]
      n298 = To Long Integer(number=w96) -> (32bit integer=w95:i32)
      n299 = Index Array(array=w100, index=w95) -> (element=w102:refnum<vi>)
      n300 = property class="Page"(reference=w102, "PageVis"=TRUE ("Page Visible")) -> ()  [unwired: 1 in, 2 out]
      n301 = property on="View Results" class="Bool"("DisabledEnum"=w74) -> ()  [unwired: 2 in, 2 out]
      n302 = property on="Run Calibration" class="Bool"("DisabledEnum"=w74) -> ()  [unwired: 2 in, 2 out]
      n303 = property on="List of All Fits" class="MCListbox (strict)"("ItemNames"=string[][] [] ("Item Names"), "Symbols Vis"=TRUE ("Visible Items:Symbols Visible")) -> ()  [unwired: 2 in, 2 out]
      n304 = property on="List of Failed Fits" class="MCListbox (strict)"("ItemNames"=string[][] [] ("Item Names")) -> ()  [unwired: 2 in, 2 out]
      n305 = while "Listener Loop: Display \"Data\" Tab" {
        shift-right: [w721] -> _
        shift-left: errorcluster {"status"=FALSE, "code"=0, "source"=""} ("error out") -> [w720]
        shift-right: [w719] -> _
        shift-left: _ -> [w718]
        stop <- w723 stop-if-true
        n306 = event shown="[2] \"List of All Fits\": Value Change" {
          selector: _ -> [_ _ _ _ _]
          dyn-events: _ -> [_ _ _ _ _]
          timeout: -1 -> [_ _ _ _ _]
          tunnel: [TRUE FALSE w738 FALSE w823] -> w723
          tunnel: [w725 w730 w742 w819 w822] -> w721
          tunnel: w720 -> [w725 w730 w737 w819 w822]
          tunnel: [w724 w727 w736 w809 w821] -> w719
          tunnel: w718 -> [w724 w727 w735 w809 w821]
          event Timeout {
            n307 = event-data() -> ()  [unwired: 1 in, 3 out]
          }
          event "List of Failed Fits": Value Change {
            n308 = event-data() -> ("NewVal"=w729:i32)  [unwired: 1 in]
            n309 = property on="List of Failed Fits" class="MCListbox (strict)"() -> ("ItemNames"=w733:string[][])  [unwired: 2 in, 2 out]
            n310 = Index Array(array=w733, index (row)=w729, index (col)=0) -> (element=w732:string)
            n311 = Decimal String To Number(string=w732) -> (number=w728:i32)  [unwired: 2 in, 1 out]
            n312 = property on="List of All Fits" class="MCListbox (strict)"("Val(Sgnl)"=w728) -> ()  [unwired: 2 in, 2 out]
          }
          event "List of All Fits": Value Change {
            n313 = event-data() -> ("OldVal"=w741:i32, "NewVal"=w739:i32)  [unwired: 1 in]
            n314 = property on="Image Data" class="Arr (strict)"() -> ("Value"=w743:T1)  [unwired: 2 in, 2 out]
            n315 = Not Equal?(x=w741, y=w739) -> (x != y?=w740:bool)
            n316 = case shown="True" w740 {
              tunnel: w743 -> [_ w802]
              tunnel: w737 -> [w746 w748]
              tunnel: [w746 w757] -> w742
              tunnel: w739 -> [_ w788]
              tunnel: [FALSE FALSE] -> w738
              tunnel: [w744 w751] -> w736
              tunnel: w735 -> [w744 w749]
              frame False {
              }
              frame True {
                w795 = T21 0 items=["Grayscale (U8)", "Grayscale (I16)", "Grayscale (SGL)", "Complex (CSG)", "RGB (U32)", "HSL (U32)", "RGB (U64)", "Grayscale (U16)"] ("Image Type")
                n317 = call "IMAQ Dispose"("Image"=w749, "error in (no error)"=w748) -> ("error out"=w747:errorcluster)  [unwired: 4 in]
                n318 = Index Array(array=w802, index=w788) -> (element=w801:T34)
                n319 = property on="Wire Diameter" class="DigNum (strict)"() -> ("Value"=w777:dbl)  [unwired: 2 in, 2 out]
                n320 = global read "PixelToMicron.vi" "PixelToMicron"() -> (w778:dbl)
                n321 = Unbundle By Name(w801) -> ("Initial Guess"=w799:cluster{"center":dbl, "reflectivity":dbl}, "parameters"=w779:T35, "errors"=w800:T35, "iterations"=w797:i32, "success?"=w796:bool, "image path"=w790:path, "image number"=w786:i32)
                n322 = Format Into String(format string="%d", initial string="Image #", w786) -> (resulting string=w781:string)  [unwired: 1 in, 1 out]
                n323 = Divide(x=w777, y=w778) -> (x/y=w766:dbl)
                n324 = Multiply(x=1.5, y=w766) -> (x*y=w773:dbl)
                n325 = Unbundle By Name(w779) -> ("center"=w775:dbl)
                n326 = Concatenate Strings("Graph of Fit for " ("string"), w781) -> (w783:string)
                n327 = Scale By Power Of 2(n=i16 -1, x=w766) -> (x*2^n=w764:dbl)
                n328 = Cluster To Array(cluster=w779) -> (array=w765:dbl[])
                n329 = Cluster To Array(cluster=w800) -> (array=w798:dbl[])
                n330 = Scale By Power Of 2(n=i16 1, x=w773) -> (x*2^n=w772:dbl)
                n331 = property on="Image" class="ImageControl"("Caption.Text"=w781) -> ()  [unwired: 2 in, 2 out]
                n332 = property on="Graph of Fit" class="XYGraph (strict)"("Caption.Text"=w783) -> ()  [unwired: 2 in, 2 out]
                n333 = Subtract(x=w775, y=w773) -> (x-y=w771:dbl)
                n334 = Bundle("Initial Guess"=w799, "parameters"=w765, "errors"=w798, "iterations"=w797, "success?"=w796) -> (→"Fit Info":T36)  [unwired: 1 in]
                n335 = To Long Integer(number=w771) -> (32bit integer=w769:i32)
                n336 = To Long Integer(number=w772) -> (32bit integer=w770:i32)
                n337 = for {
                  N: w770 -> [_]
                  tunnel: w769 -> [w807]
                  tunnel: [w806] -> w768 mode=indexing
                  i -> [w808]
                  n338 = Add(x=w807, y=w808) -> (x+y=w806:i32)
                }
                n339 = Strip Path(path=w790) -> (name=w791:string)  [unwired: 1 out]
                n340 = Search/Split String(string=w791, search string/char (-)=".") -> (substring before match=w793:string)  [unwired: 1 in, 2 out]
                n341 = To Double Precision Float(number=w768) -> (double precision float=w755:dbl[])
                n342 = Build Array (concatenate)(w765, w764) -> (w754:dbl[])
                n343 = call "IMAQ Create"("Image Name"=w793, "Image Type"=w795, "error in (no error)"=w747) -> ("New Image"=w792:T7, "error out"=w789:errorcluster)  [unwired: 2 in]
                n344 = for {
                  tunnel: [w805] -> w756 mode=indexing
                  tunnel: w755 -> [w804] mode=indexing
                  tunnel: w754 -> [w803]
                  n345 = call "JoelReflectivityModel.vi"("Parameters"=w803, "x"=w804) -> ("y"=w805:dbl)  [unwired: 8 in, 1 out]
                }
                n346 = call "IMAQ ReadFile"("File Path"=w790, "error in (no error)"=w789, "Image"=w792) -> ("error out"=w780:errorcluster, "Image Out"=w751:T7)  [unwired: 4 in, 3 out]
                "Image" <- w751
                n347 = call "GetImageData.vi"("error in (no error)"=w780, "Image"=w751) -> ("error out"=w757:errorcluster, "Array"=w753:dbl[])  [unwired: 7 in]
                n348 = call "SimpleVariance.vi"("X"=w753) -> ("variance"=w752:dbl[])  [unwired: 1 in, 1 out]
                n349 = Array Subset(array=w752, index=w769, length=w770) -> (w762:dbl[])
                n350 = Bundle(w755, w762) -> (w760:cluster{dbl[], dbl[]})  [unwired: 1 in]
                n351 = Select(t=dbl[] [], s=w757, f=w756) -> (s? t:f=w758:dbl[])
                n352 = Bundle(w755, "t"=w758) -> (w761:cluster{dbl[], "t":dbl[]})  [unwired: 1 in]
                n353 = Build Array(w760, w761) -> (w763:cluster{dbl[], "t":dbl[]}[])
                n354 = property on="Graph of Fit" class="XYGraph (strict)"("Value"=w763) -> ()  [unwired: 2 in, 2 out]
              }
            }
            "Image Display Error" <- w737
          }
          event "Image Data": Value Change {
            n355 = event-data() -> ("OldVal"=w815:T1, "NewVal"=w818:T1)  [unwired: 1 in]
            n356 = property on="List of All Fits" class="MCListbox (strict)"() -> ("Value"=w816:i32)  [unwired: 2 in, 2 out]
            n357 = Increment(x=w816) -> (x+1=w811:i32)
            n358 = Array Size(array=w815) -> (size(s)=w814:i32)
            n359 = Equal?(x=w811, y=w814) -> (x = y?=w813:bool)
            n360 = Array Size(array=w818) -> (size(s)=w812:i32)
            n361 = Decrement(x=w812) -> (x-1=w810:i32)
            n362 = case shown="True" w813 {
              tunnel: w810 -> [_ w820]
              frame False {
              }
              frame True {
                n363 = property on="List of All Fits" class="MCListbox (strict)"("Val(Sgnl)"=w820) -> ()  [unwired: 2 in, 2 out]
              }
            }
          }
          event "Quit": Value Change {
            n364 = event-data() -> ("NewVal"=w823:bool)  [unwired: 1 in]
          }
        }
      }
    }
  }
  n365 = while "Show/Hide Troubleshooting Tab" {
    stop <- w825 stop-if-true
    n366 = event shown="[2] \"error tab\": Value Change" {
      selector: _ -> [_ _ _]
      dyn-events: _ -> [_ _ _]
      timeout: -1 -> [_ _ _]
      tunnel: [TRUE ("NewVal") w827 FALSE ("NewVal")] -> w825
      event Timeout {
        n367 = event-data() -> ()  [unwired: 1 in, 1 out]
      }
      event "Quit": Value Change {
        n368 = event-data() -> ("NewVal"=w827:bool)  [unwired: 1 in]
      }
      event "error tab": Value Change {
        n369 = event-data() -> ("NewVal"=w830:bool)  [unwired: 1 in]
        n370 = property on="Tab Control" class="TabCtl (strict)"() -> ("Pages"=w832:refnum<vi>[])  [unwired: 2 in, 2 out]
        n371 = Index Array(array=w832, index=3) -> (element=w831:refnum<vi>)
        n372 = property class="Page"(reference=w831, "PageVis"=w830) -> ()  [unwired: 1 in, 2 out]
      }
    }
  }
  n373 = control-ref of="Y position"() -> (w5:refnum<vi>)
  n374 = control-ref of="Z position"() -> (w4:refnum<vi>)
  n375 = Build Array(w5, w4) -> (w2:refnum<vi>[])
  n376 = Current VI's Path() -> (path=w3:path)
  n377 = call "LoadFromConfig.vi"("Array"=w2, "Section"="pos", "VI Path"=w3) -> ()
